vi "path_plan.vi"(4 "Node2":string="C400D1", 5 "z":dbl=420.0, 6 "y":dbl=7988.0, 7 "x":dbl=8250.0) -> (0 "Path坐标数组":dbl[][](array[numeric]), 1 "Dis 2":dbl, 2 "Area 3":string[](array[string]), 3 "Path 2":string[](array[string]))   [LabVIEW 2014]
uses:
  <vilib>/Utility/importsl/GetValueByPointer/datatype.ctl
  <vilib>/Utility/importsl/GetValueByPointer/GetValueByPointer.xnode
  path_plan6.dll
  get_co.dll
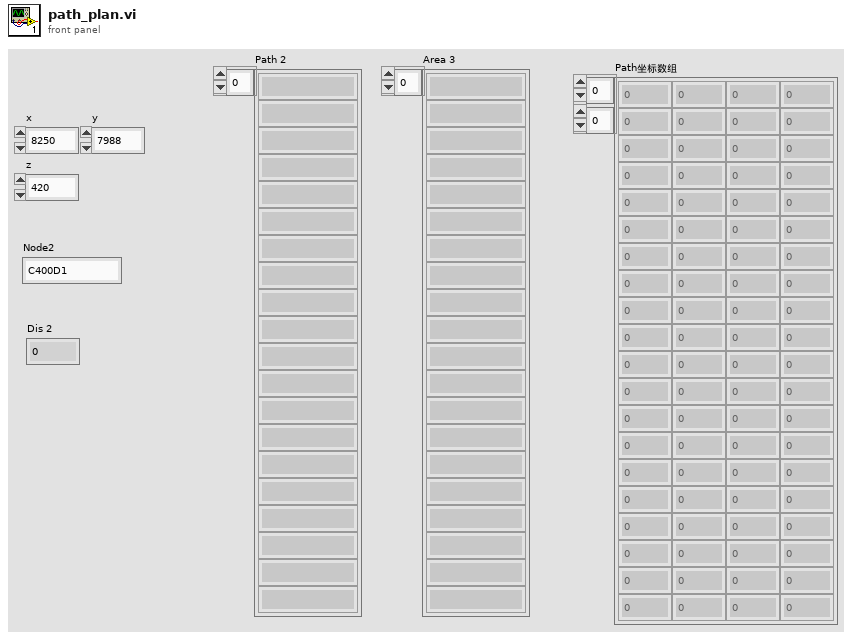
[diagram p1: front panel]
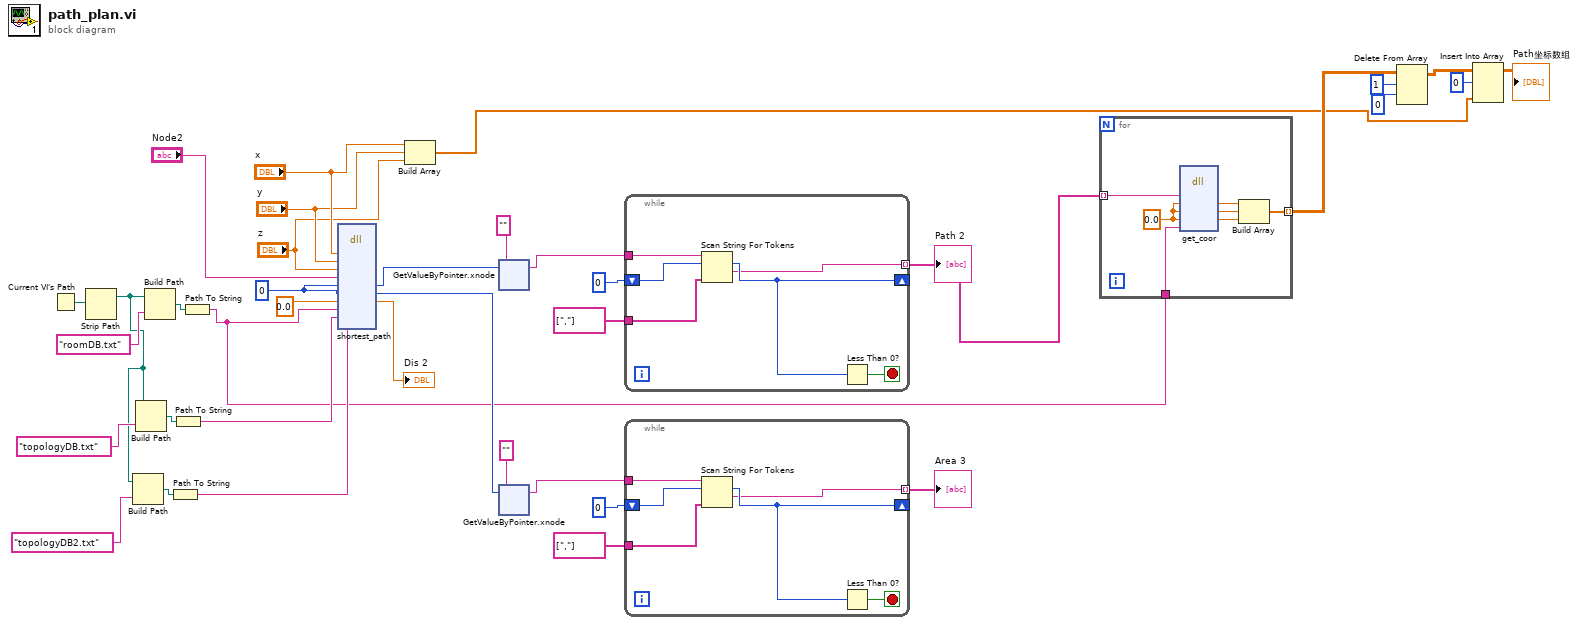
[diagram p0: block diagram]
diagram:
  w25 = 0 ("Path")
  n1 = Current VI's Path() -> (path=w11:path)
  n2 = Strip Path(path=w11) -> (stripped path=w2:path)  [unwired: 1 out]
  n3 = Build Path(base path=w2, name or relative path="topologyDB2.txt" ("roomDB")) -> (appended path=w7:path)
  n4 = Build Path(base path=w2, name or relative path="topologyDB.txt" ("roomDB")) -> (appended path=w8:path)
  n5 = Build Path(base path=w2, name or relative path="roomDB.txt" ("roomDB")) -> (appended path=w10:path)
  n6 = Path To String(path=w7) -> (string=w3:string)
  n7 = Path To String(path=w8) -> (string=w4:string)
  n8 = Path To String(path=w10) -> (string=w1:string)
  n9 = dll-call lib="E:/labview/1511/zsControlSystem2.0/FromOtherProject/FromLXY/speech/path_plan6.dll" fn="shortest_path"("X"="x", "Y"="y", "Z"="z", "Node2"="Node2", "Path"=w25, "Area"=w25, "Dis"=0.0, "roomDB"=w1, "topologyDB"=w4, "topologyDB2"=w3) -> ("Path"=w28:i32, "Area"=w26:i32, "Dis"=→"Dis 2":dbl)  [unwired: 11 in, 2 out]
  n10 = Build Array("x", "y", "z") -> (w13:dbl[])
  n11 = xnode "GetValueByPointer.xnode"("Pointer"=w28, "InputType"="") -> ("Output"=w34:string)  [unwired: 2 in, 1 out]
  n12 = xnode "GetValueByPointer.xnode"("Pointer"=w26, "InputType"="") -> ("Output"=w29:string)  [unwired: 2 in, 1 out]
  n13 = while {
    shift-right: [w41] -> _
    shift-left: 0 -> [w43]
    tunnel: [w40] -> w23 mode=indexing
    tunnel: string[] [","] ("分隔符(\\s,\\t,\\r,\\n)") -> [w39]
    tunnel: w34 -> [w38]
    stop <- w42 stop-if-true
    n14 = Scan String For Tokens(6:w39, 8:w43, 9:w38) -> (1:w40:string, 2:w41:i32)  [unwired: 3 in, 2 out]
    n15 = Less Than 0?(x=w41) -> (x < 0?=w42:bool)
  }
  "Path 2" <- w23
  n16 = while {
    shift-right: [w47] -> _
    shift-left: 0 -> [w49]
    tunnel: [w46] -> w31 mode=indexing
    tunnel: string[] [","] ("分隔符(\\s,\\t,\\r,\\n)") -> [w45]
    tunnel: w29 -> [w44]
    stop <- w48 stop-if-true
    n17 = Scan String For Tokens(6:w45, 8:w49, 9:w44) -> (1:w46:string, 2:w47:i32)  [unwired: 3 in, 2 out]
    n18 = Less Than 0?(x=w47) -> (x < 0?=w48:bool)
  }
  "Area 3" <- w31
  n19 = for {
    tunnel: w23 -> [w52] mode=indexing
    tunnel: [w51] -> w18 mode=indexing
    tunnel: w1 -> [w50]
    w56 = 0.0 ("参数2")
    n20 = dll-call lib="E:/labview/1511/zsControlSystem2.0/FromOtherProject/FromLXY/speech/get_co.dll" fn="get_coor"("Node"=w52, "X"=w56, "Y"=w56, "Z"=w56, "Room"=w50) -> ("X"=w55:dbl, "Y"=w54:dbl, "Z"=w53:dbl)  [unwired: 6 in, 2 out]
    n21 = Build Array(w55, w54, w53) -> (w51:dbl[])
  }
  n22 = Delete From Array(array=w18, length=1 ("长度"), index (row)=0 ("索引 (行)")) -> (array with subset deleted=w15:dbl[][])  [unwired: 1 in, 1 out]
  n23 = Insert Into Array(array=w15, index (row)=0 ("索引 (行)"), new element=w13) -> (→"Path坐标数组":dbl[][])  [unwired: 1 in]
